vi "percentage_input.vi"(1 "input":dbl[](array[numeric])) -> (0 "desired_output":dbl[](array[numeric]))   [LabVIEW 2021, in "CALIBRATION.lvlib"]
uses:
  CALIBRATION.lvlib
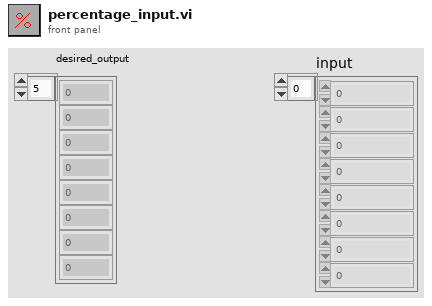
[diagram p1: front panel]
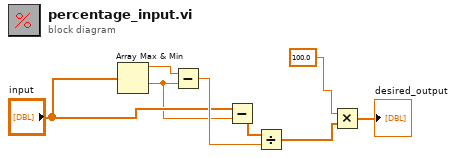
[diagram p0: block diagram]
diagram:
  n1 = Array Max & Min(array="input") -> (max value=w5:dbl, min value=w1:dbl)  [unwired: 2 out]
  n2 = Subtract(x=w5, y=w1) -> (x-y=w4:dbl)
  n3 = Subtract(x="input", y=w1) -> (x-y=w3:dbl[])
  n4 = Divide(x=w3, y=w4) -> (x/y=w8:dbl[])
  n5 = Multiply(x=100.0, y=w8) -> (x*y=→"desired_output":dbl[])
